vi "Set Output.vi"(4 "Offset":dbl min=-3.0 max=4.0 format="%.2f", 5 "Load":bool, 6 "Amplitude":dbl=1.0 min=-3.0 max=4.0 format="%.2f", 7 "Polarity":bool, 8 "error in (no error)":errorcluster, 9 "Output Level":T2, 10 "Channel":T1, 11 "VISA Refnum in":refnum<visa-resource-name>) -> (0 "error out":errorcluster)   [LabVIEW 2012, in "SRS_DG535_Lib.lvlib"]
uses:
  SRS_DG535_Lib.lvlib
  Command/DG535_Output.ctl
  Command/DG535_Channel.ctl
panel:
  out "output string":string
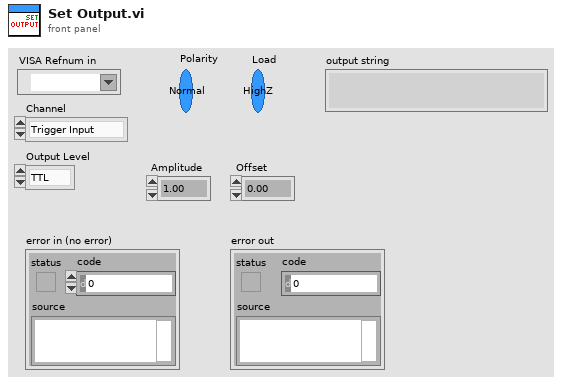
[diagram p1: front panel]
types:
  T1 = typedef "SRS_DG535_Lib.lvlib/DG535_Channel.ctl" = enum16{"Trigger Input", "T0 Output", "A Output", "B Output", "AB Output", "C Output", "D Output", "CD Output", "NULL"}
  T2 = typedef "SRS_DG535_Lib.lvlib/DG535_Output.ctl" = enum16{"TTL", "NIM", "ECL", "Variable"}
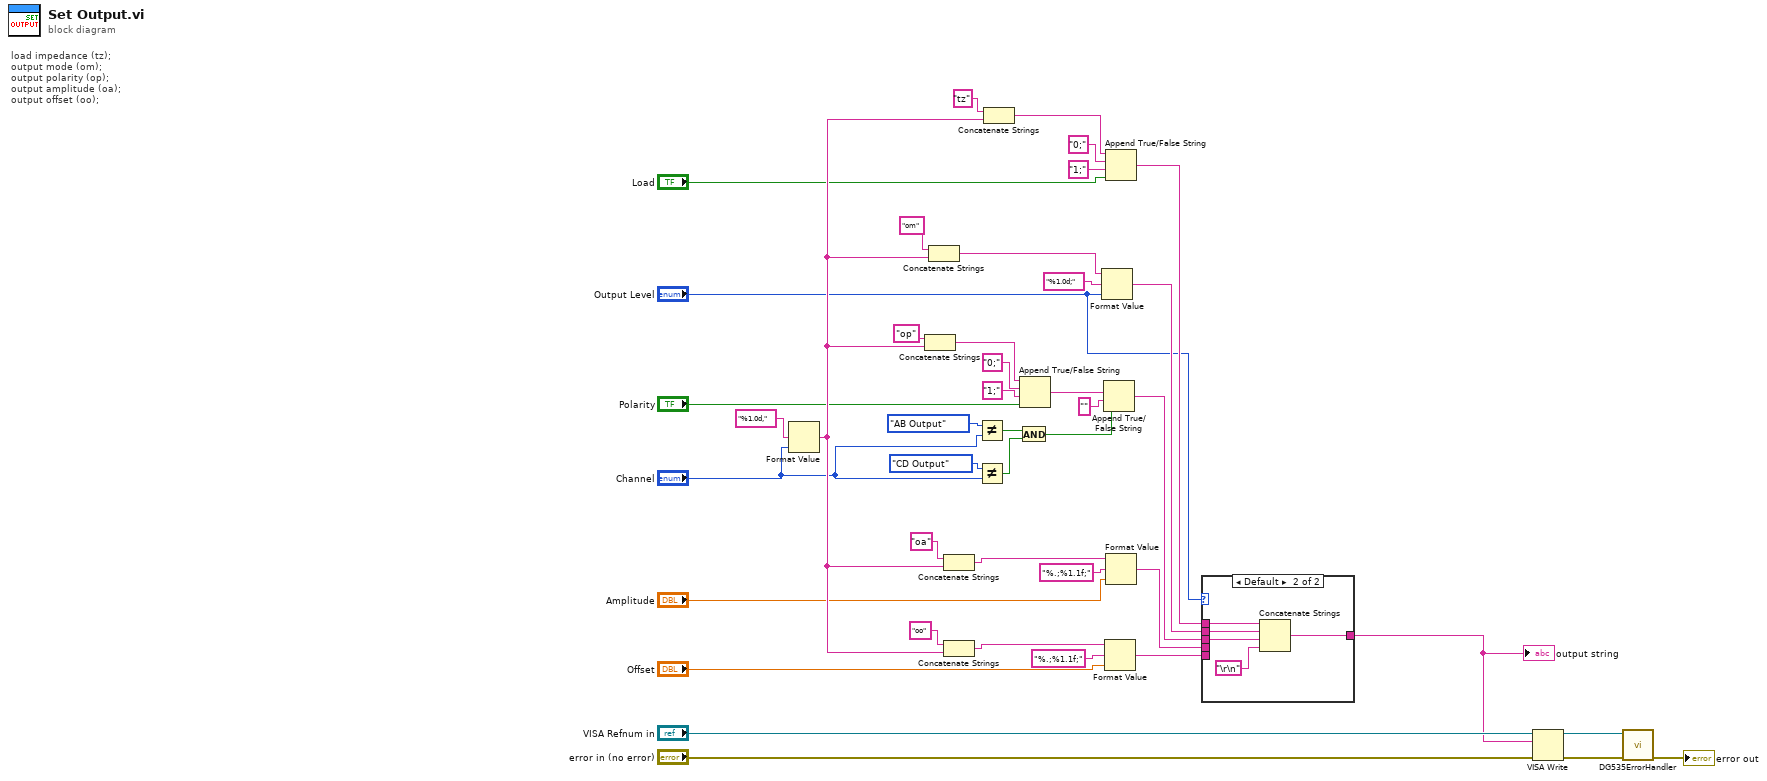
[diagram p0: block diagram]
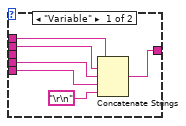
[diagram p2: hidden frame]
diagram:
  # "load impedance (tz);\noutput mode (om);\noutput polarity (op);\noutput amplitude (oa);\noutput offset (oo);"
  n1 = Format Value(format string="%1.0d,", value (0)="Channel") -> (output string=w26:string)  [unwired: 1 in]
  n2 = Concatenate Strings("op", w26) -> (w40:string)
  n3 = Concatenate Strings("om", w26) -> (w39:string)
  n4 = Concatenate Strings("oa", w26) -> (w41:string)
  n5 = Concatenate Strings("oo", w26) -> (w18:string)
  n6 = Not Equal?(x=DG535_Channel."AB Output", y="Channel") -> (x != y?=w28:bool)
  n7 = Not Equal?(x=DG535_Channel."CD Output", y="Channel") -> (x != y?=w27:bool)
  n8 = Concatenate Strings("tz", w26) -> (w38:string)
  n9 = And(x=w28, y=w27) -> (x .and. y?=w37:bool)
  n10 = Append True/False String(1:"Polarity", 2:"1;", 3:"0;", 4:w40) -> (0:w16:string)
  n11 = Format Value(string ("")=w39, format string="%1.0d;", value (0)="Output Level") -> (output string=w9:string)
  n12 = Append True/False String(1:w37, 2:"", 3:w16) -> (0:w8:string)  [unwired: 1 in]
  n13 = Format Value(string ("")=w18, format string="%.;%1.1f;", value (0)="Offset") -> (output string=w6:string)
  n14 = Append True/False String(1:"Load", 2:"1;", 3:"0;", 4:w38) -> (0:w10:string)
  n15 = Format Value(string ("")=w41, format string="%.;%1.1f;", value (0)="Amplitude") -> (output string=w7:string)
  n16 = case shown="Default" "Output Level" {
    tunnel: w10 -> [w49 w54]
    tunnel: w9 -> [w48 w53]
    tunnel: w8 -> [_ w52]
    tunnel: w7 -> [w47 _]
    tunnel: w6 -> [w46 _]
    tunnel: [w44 w51] -> w1
    frame "Variable" {
      n17 = Concatenate Strings(w49, w48, w47, w46, "\r\n") -> (w44:string)
    }
    frame Default {
      n18 = Concatenate Strings(w54, w53, w52, "\r\n") -> (w51:string)
    }
  }
  "output string" <- w1
  n19 = VISA Write(VISA resource name="VISA Refnum in", write buffer=w1, error in (no error)="error in (no error)") -> (VISA resource name out=w3:refnum<visa-resource-name>, error out=w5:errorcluster)  [unwired: 1 out]
  n20 = call "DG535ErrorHandler.vi"("error in"=w5, "VISA resource name"=w3) -> ("error out"=→"error out":errorcluster)  [unwired: 7 in, 2 out]
